vi "FlatToRichrfcontrol_SetRFDCCenterFrequencyRequest.vi"(5 "OutputClusterType":T1, 11 "InputCluster":T3) -> (3 "OutputCluster":T1)   [LabVIEW 2024, in "FlexSDR_gRPC_client.lvlib"]
uses:
  rfcontrol_SetRFDCCenterFrequencyRequest_Flat.ctl
  rfcontrol_RFDC.ctl
  rfcontrol_SetRFDCCenterFrequencyRequest.ctl
  FlexSDR_gRPC_client.lvlib
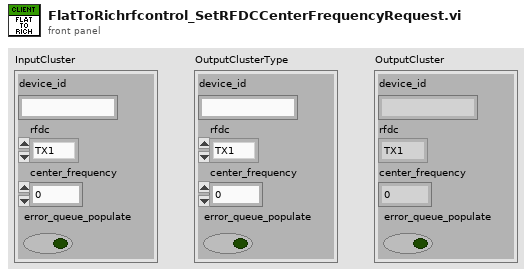
[diagram p1: front panel]
types:
  T1 = typedef "FlexSDR_gRPC_client.lvlib/rfcontrol_SetRFDCCenterFrequencyRequest.ctl" = cluster{"device_id":string, "rfdc":T2, "center_frequency":dbl, "error_queue_populate":bool}
  T2 = typedef "FlexSDR_gRPC_client.lvlib/rfcontrol_RFDC.ctl" = enum32{"TX1", "TX2", "TX3", "TX4", "TX5", "TX6", "TX7", "TX8", "RX1", "RX2", "RX3", "RX4", "RX5", "RX6", "RX7", "RX8", "WRX1", "WRX2"}
  T3 = typedef "FlexSDR_gRPC_client.lvlib/rfcontrol_SetRFDCCenterFrequencyRequest_Flat.ctl" = cluster{"device_id":string, "rfdc":T2, "center_frequency":dbl, "error_queue_populate":bool}
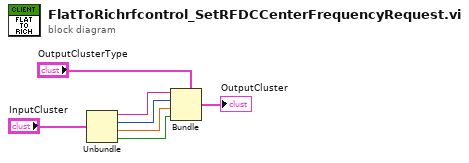
[diagram p0: block diagram]
diagram:
  n1 = Unbundle "Unbundle"("InputCluster") -> ("device_id"=w4:string, "rfdc"=w3:T2, "center_frequency"=w2:dbl, "error_queue_populate"=w1:bool)
  n2 = Bundle "Bundle"(cluster="OutputClusterType", "device_id"=w4, "rfdc"=w3, "center_frequency"=w2, "error_queue_populate"=w1) -> (→"OutputCluster":T1)
